vi "Write Icon Text.vi"(8 "error in (no error)":errorcluster, 10 "Icon Text":string, 11 "MGI_TrayIcon in":refnum<class "MGI_TrayIcon.lvclass">) -> (0 "error out":errorcluster, 3 "MGI_TrayIcon out":refnum<class "MGI_TrayIcon.lvclass">)   [LabVIEW 2016, in "MGI_TrayIcon.lvclass"]
doc: "Authored by Derek E. Trepanier\nsupport@mooregoodideas.com\nwww.mooregoodideas.com\n\nCopyright (c) 2012, Moore Good Ideas, Inc.\n\nAll rights reserved.\n\nRedistribution and use in source and binary forms, with or without modification, are permitted provided that the following conditions are met:\n\n * Redistributions of source code must retain the above copyright notice, this list of conditions and the following disclaimer.\n * Redistributions in binary form must reproduce the above copyright notice, this list of conditions and the following disclaimer in the documentation and/or other materials provided with the distribution.\n * Neither the name of Moore Good Ideas, Inc. nor the names of its contributors may be used to endorse or promote products derived from this software without specific prior written permission.\n\nTHIS SOFTWARE IS PROVIDED BY THE COPYRIGHT HOLDERS AND CONTRIBUTORS \"AS IS\" AND ANY EXPRESS OR IMPLIED WARRANTIES, INCLUDING, BUT NOT LIMITED TO, THE IMPLIED WARRANTIES OF MERCHANTABILITY AND FITNESS FOR A PARTICULAR PURPOSE ARE DISCLAIMED. IN NO EVENT SHALL THE COPYRIGHT OWNER OR CONTRIBUTORS BE LIABLE FOR ANY DIRECT, INDIRECT, INCIDENTAL, SPECIAL, EXEMPLARY, OR CONSEQUENTIAL DAMAGES (INCLUDING, BUT NOT LIMITED TO, PROCUREMENT OF SUBSTITUTE GOODS OR SERVICES; LOSS OF USE, DATA, OR PROFITS; OR BUSINESS INTERRUPTION) HOWEVER CAUSED AND ON ANY THEORY OF LIABILITY, WHETHER IN CONTRACT, STRICT LIABILITY, OR TORT (INCLUDING NEGLIGENCE OR OTHERWISE) ARISING IN ANY WAY OUT OF THE USE OF THIS SOFTWARE, EVEN IF ADVISED OF THE POSSIBILITY OF SUCH DAMAGE."
uses:
  <userlib>/_MGI/Menu Building/MenuTypes/TrayIcon/MGI_TrayIcon.lvclass
  <userlib>/_MGI/Menu Building/MenuTypes/TrayIcon/MGI_TrayIcon.lvclass/MGI_TrayIcon.ctl
  System.Windows.Forms
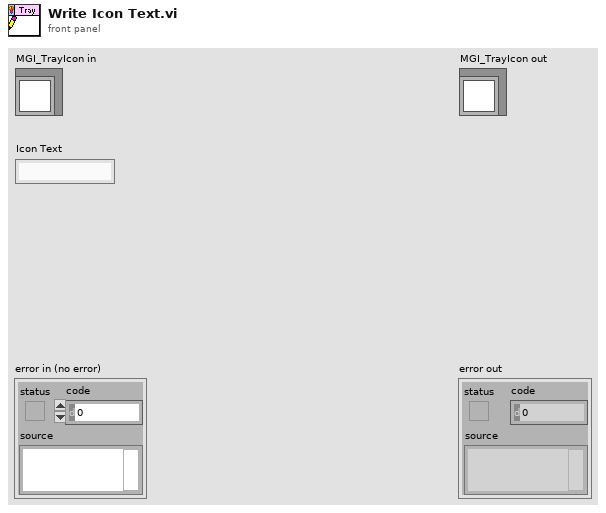
[diagram p1: front panel]
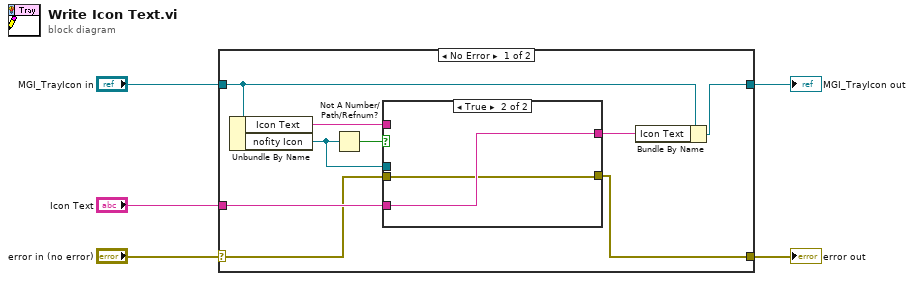
[diagram p0: block diagram]
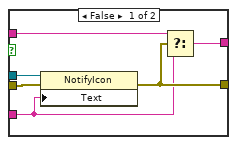
[diagram p2: hidden frame]
diagram:
  n1 = case shown="No Error" "error in (no error)" {
    selector: "error in (no error)" -> [w7 w23]
    tunnel: [w6 w23] -> w4
    tunnel: [w14 w24] -> w2
    tunnel: "MGI_TrayIcon in" -> [w13 w24]
    tunnel: "Icon Text" -> [w8 _]
    frame No Error {
      n2 = Unbundle By Name(w13) -> ("Icon Text"=w11:string, "nofity Icon"=w10:refnum<k24>)
      n3 = Not A Number/Path/Refnum?(number/path/refnum=w10) -> (NaN/Path/Refnum?=w12:bool)
      n4 = case shown="True" w12 {
        tunnel: w11 -> [w16 _]
        tunnel: w10 -> [w20 _]
        tunnel: [w17 w22] -> w9
        tunnel: w8 -> [w15 w22]
        tunnel: w7 -> [w19 w21]
        tunnel: [w18 w21] -> w6
        frame False {
          n5 = property class="NotifyIcon"(reference=w20, error in=w19, "Text"=w15) -> (error out=w18:errorcluster)  [unwired: 1 out]
          n6 = Select(t=w16, s=w18, f=w15) -> (s? t:f=w17:string)
        }
        frame True {
        }
      }
      n7 = Bundle By Name(cluster=w13, "Icon Text"=w9) -> (w14:refnum<class "MGI_TrayIcon.lvclass">)
    }
    frame Error {
    }
  }
  "error out" <- w4
  "MGI_TrayIcon out" <- w2
